vi "Pacemaker ASIC Test_Config Globals.vi"() -> ()   [LabVIEW 2016]
panel:
  in  "software version 2":string="build  2097"
  in  "software version 1":string="ASIC Test  V0.10.0.1"
  out "uut  note":string="IC_all"
  in  "id strings":string[][](table)
  out "note":string
  out "data time":string="20121102_163200"
  out "uut  sn":string="29A"
  out "uut version":string="03A"
  out "uut pn":string="MC20"
  in  "Shunt":T1={"Ib Vol"=1.0, "Ib Cur"=1e-08, "Ibat Vol"=0.007765, "Ibat Cur"=1e-06, "Load Vrega Vol"=-1.0, "Load Vrega Cur"=1e-05, "Load Vregd Vol"=-1.0, "Load Vregd Cur"=0.0002, "Load Vha Vol"=-1.0, "Load Vha Cur"=0.0002} {"Load Vha Cur" format="%#_6p"; "Load Vregd Cur" format="%#_6p"; "Load Vrega Cur" format="%#_6p"; "Ibat Cur" format="%#_6p"; "Ibat Vol" format="%#_6p"; "Ib Cur" format="%#_6p"; "Ib Vol" format="%#_6p"}
  out "TableReg":string[][](table)=[["Function_Name", "Bit_Name", "Data[B]", ""], ["System Control Register", "CPUOk", "0", ""], ["System Control Register", "RDSMASK", "0", ""], ["System Control Register", "LPWMASK", "0", ""], ["System Control Register", "TPSLEEP", "0", ""], ["System Control Register", "VUR", "0", ""], ["System Control Register", "VUT", "1", ""], ["System Control Register", "AUR", "0", ""], ["System Control Register", "AUT", "1", ""], ["Atrial Pulse Dutation Control Register", "ABILUNISEL", "1", ""], ["Atrial Pulse Dutation Control Register", "ARCHG[2]", "1", ""], ["Atrial Pulse Dutation Control Register", "ARCHG[1]", "0", ""], ["Atrial Pulse Dutation Control Register", "ARCHG[0]", "1", ""], ["Atrial Pulse Dutation Control Register", "APW[3]", "1", ""], ["Atrial Pulse Dutation Control Register", "APW[2]", "0", ""], ["Atrial Pulse Dutation Control Register", "APW[1]", "0", ""], ["Atrial Pulse Dutation Control Register", "APW[0]", "0", ""], ["Atrial Pace Amplitude Control Register", "APUMPGN[1]", "1", ""], ["Atrial Pace Amplitude Control Register", "APUMPGN[0]", "0", ""], ["Atrial Pace Amplitude Control Register", "APAMP[5]", "1", ""], ["Atrial Pace Amplitude Control Register", "APAMP[4]", "0", ""], ["Atrial Pace Amplitude Control Register", "APAMP[3]", "1", ""], ["Atrial Pace Amplitude Control Register", "APAMP[2]", "0", ""], ["Atrial Pace Amplitude Control Register", "APAMP[1]", "0", ""], ["Atrial Pace Amplitude Control Register", "APAMP[0]", "0", ""], ["Ventricular Pulse Duration Control Register", "VBILUNISEL", "1", ""], ["Ventricular Pulse Duration Control Register", "VRCHG[2]", "1", ""], ["Ventricular Pulse Duration Control Register", "VRCHG[1]", "0", ""], ["Ventricular Pulse Duration Control Register", "VRCHG[0]", "1", ""], ["Ventricular Pulse Duration Control Register", "VPW[3]", "1", ""], ["Ventricular Pulse Duration Control Register", "VPW[2]", "0", ""], ["Ventricular Pulse Duration Control Register", "VPW[1]", "0", ""], ["Ventricular Pulse Duration Control Register", "VPW[0]", "0", ""], ["Ventricular Pace Amplitude Control Register", "VPUMPGN[1]", "1", ""], ["Ventricular Pace Amplitude Control Register", "VPUMPGN[0]", "0", ""], ["Ventricular Pace Amplitude Control Register", "VPAMP[5]", "1", ""], ["Ventricular Pace Amplitude Control Register", "VPAMP[4]", "0", ""], ["Ventricular Pace Amplitude Control Register", "VPAMP[3]", "1", ""], ["Ventricular Pace Amplitude Control Register", "VPAMP[2]", "0", ""], ["Ventricular Pace Amplitude Control Register", "VPAMP[1]", "0", ""], ["Ventricular Pace Amplitude Control Register", "VPAMP[0]", "0", ""], ["Blank/Mask Control Register", "AAIFLG", "0", ""], ["Blank/Mask Control Register", "PVAB[4]", "0", ""], ["Blank/Mask Control Register", "PVAB[3]", "1", ""], ["Blank/Mask Control Register", "PVAB[2]", "0", ""], ["Blank/Mask Control Register", "PVAB[1]", "0", ""], ["Blank/Mask Control Register", "PVAB[0]", "1", ""], ["Blank/Mask Control Register", "OBLANK[1]", "1", ""], ["Blank/Mask Control Register", "OBLANK[0]", "1", ""], ["Atrial Sensitivity Control Register", "Spare", "0", ""], ["Atrial Sensitivity Control Register", "ASGN[1]", "1", ""], ["Atrial Sensitivity Control Register", "ASGN[0]", "1", ""], ["Atrial Sensitivity Control Register", "AS[4]", "0", ""], ["Atrial Sensitivity Control Register", "AS[3]", "1", ""], ["Atrial Sensitivity Control Register", "AS[2]", "0", ""], ["Atrial Sensitivity Control Register", "AS[1]", "0", ""], ["Atrial Sensitivity Control Register", "AS[0]", "1", ""], ["Ventricular Sensitivity Control Register", "Spare", "0", ""], ["Ventricular Sensitivity Control Register", "VSGN[1]", "0", ""], ["Ventricular Sensitivity Control Register", "VSGN[0]", "1", ""], ["Ventricular Sensitivity Control Register", "VS[4]", "0", ""], ["Ventricular Sensitivity Control Register", "VS[3]", "1", ""], ["Ventricular Sensitivity Control Register", "VS[2]", "1", ""], ["Ventricular Sensitivity Control Register", "VS[1]", "0", ""], ["Ventricular Sensitivity Control Register", "VS[0]", "1", ""], ["Measure Request Register", "Spare", "0", ""], ["Measure Request Register", "TPUMPEN", "0", ""], ["Measure Request Register", "EGMFS", "0", ""], ["Measure Request Register", "EGMREQ[1]", "0", ""], ["Measure Request Register", "EGMREQ[0]", "0", ""], ["Measure Request Register", "MREQ[2]", "0", ""], ["Measure Request Register", "MREQ[1]", "0", ""], ["Measure Request Register", "MREQ[0]", "0", ""], ["Measurement Result Register 1", "MRESULT1[7]", "0", ""], ["Measurement Result Register 1", "MRESULT1[6]", "0", ""], ["Measurement Result Register 1", "MRESULT1[5]", "0", ""], ["Measurement Result Register 1", "MRESULT1[4]", "0", ""], ["Measurement Result Register 1", "MRESULT1[3]", "0", ""], ["Measurement Result Register 1", "MRESULT1[2]", "0", ""], ["Measurement Result Register 1", "MRESULT1[1]", "0", ""], ["Measurement Result Register 1", "MRESULT1[0]", "0", ""], ["Measurement Result Register 2", "MRESULT2[7]", "0", ""], ["Measurement Result Register 2", "MRESULT2[6]", "0", ""], ["Measurement Result Register 2", "MRESULT2[5]", "0", ""], ["Measurement Result Register 2", "MRESULT2[4]", "0", ""], ["Measurement Result Register 2", "MRESULT2[3]", "0", ""], ["Measurement Result Register 2", "MRESULT2[2]", "0", ""], ["Measurement Result Register 2", "MRESULT2[1]", "0", ""], ["Measurement Result Register 2", "MRESULT2[0]", "0", ""], ["Telemetry Downlink Data Length Register", "Spare", "0", ""], ["Telemetry Downlink Data Length Register", "Spare", "0", ""], ["Telemetry Downlink Data Length Register", "RFDLEN2CPU[5]", "0", ""], ["Telemetry Downlink Data Length Register", "RFDLEN2CPU[4]", "0", ""], ["Telemetry Downlink Data Length Register", "RFDLEN2CPU[3]", "0", ""], ["Telemetry Downlink Data Length Register", "RFDLEN2CPU[2]", "0", ""], ["Telemetry Downlink Data Length Register", "RFDLEN2CPU[1]", "0", ""], ["Telemetry Downlink Data Length Register", "RFDLEN2CPU[0]", "0", ""], ["Telemetry Marker Low Byte Data Register", "MARKER2RF[7]", "0", ""], ["Telemetry Marker Low Byte Data Register", "MARKER2RF[6]", "0", ""], ["Telemetry Marker Low Byte Data Register", "MARKER2RF[5]", "0", ""], ["Telemetry Marker Low Byte Data Register", "MARKER2RF[4]", "0", ""], ["Telemetry Marker Low Byte Data Register", "MARKER2RF[3]", "0", ""], ["Telemetry Marker Low Byte Data Register", "MARKER2RF[2]", "0", ""], ["Telemetry Marker Low Byte Data Register", "MARKER2RF[1]", "0", ""], ["Telemetry Marker Low Byte Data Register", "MARKER2RF[0]", "0", ""], ["Telemetry Marker High Byte Data Register", "MARKER2RF[15]", "0", ""], ["Telemetry Marker High Byte Data Register", "MARKER2RF[14]", "0", ""], ["Telemetry Marker High Byte Data Register", "MARKER2RF[13]", "0", ""], ["Telemetry Marker High Byte Data Register", "MARKER2RF[12]", "0", ""], ["Telemetry Marker High Byte Data Register", "MARKER2RF[11]", "0", ""], ["Telemetry Marker High Byte Data Register", "MARKER2RF[10]", "0", ""], ["Telemetry Marker High Byte Data Register", "MARKER2RF[9]", "0", ""], ["Telemetry Marker High Byte Data Register", "MARKER2RF[8]", "0", ""], ["Telemetry Handshake Data Register", "RSW", "0", ""], ["Telemetry Handshake Data Register", "HSOK", "0", ""], ["Telemetry Handshake Data Register", "TPINSS", "0", ""], ["Telemetry Handshake Data Register", "TBD[4]", "0", ""], ["Telemetry Handshake Data Register", "TBD[3]", "0", ""], ["Telemetry Handshake Data Register", "TBD[2]", "0", ""], ["Telemetry Handshake Data Register", "TBD[1]", "0", ""], ["Telemetry Handshake Data Register", "TBD[0]", "0", ""], ["Telemetry Session ID Register", "SID2RF", "0", ""], ["Telemetry Session ID Register", "SID2RF", "0", ""], ["Telemetry Session ID Register", "SID2RF", "0", ""], ["Telemetry Session ID Register", "SID2RF", "0", ""], ["Telemetry Session ID Register", "SID2RF", "0", ""], ["Telemetry Session ID Register", "SID2RF", "0", ""], ["Telemetry Session ID Register", "SID2RF", "0", ""], ["Telemetry Session ID Register", "SID2RF", "0", ""], ["BIR Result Low Register", "BIRRESU[7]", "0", ""], ["BIR Result Low Register", "BIRRESU[6]", "0", ""], ["BIR Result Low Register", "BIRRESU[5]", "0", ""], ["BIR Result Low Register", "BIRRESU[4]", "0", ""], ["BIR Result Low Register", "BIRRESU[3]", "0", ""], ["BIR Result Low Register", "BIRRESU[2]", "0", ""], ["BIR Result Low Register", "BIRRESU[1]", "0", ""], ["BIR Result Low Register", "BIRRESU[0]", "0", ""], ["BIR Result High Register", "Spare", "0", ""], ["BIR Result High Register", "Spare", "0", ""], ["BIR Result High Register", "Spare", "0", ""], ["BIR Result High Register", "Spare", "0", ""], ["BIR Result High Register", "Spare", "0", ""], ["BIR Result High Register", "Spare", "0", ""], ["BIR Result High Register", "BIRRESU[9]", "0", ""], ["BIR Result High Register", "BIRRESU[8]", "0", ""], ["Pump Time Low Register", "TPUMP[7]", "0", ""], ["Pump Time Low Register", "TPUMP[6]", "0", ""], ["Pump Time Low Register", "TPUMP[5]", "0", ""], ["Pump Time Low Register", "TPUMP[4]", "0", ""], ["Pump Time Low Register", "TPUMP[3]", "0", ""], ["Pump Time Low Register", "TPUMP[2]", "0", ""], ["Pump Time Low Register", "TPUMP[1]", "0", ""], ["Pump Time Low Register", "TPUMP[0]", "0", ""], ["Pump Time High Register", "TPUMP[15]", "0", ""], ["Pump Time High Register", "TPUMP[14]", "0", ""], ["Pump Time High Register", "TPUMP[13]", "0", ""], ["Pump Time High Register", "TPUMP[12]", "0", ""], ["Pump Time High Register", "TPUMP[11]", "0", ""], ["Pump Time High Register", "TPUMP[10]", "0", ""], ["Pump Time High Register", "TPUMP[9]", "0", ""], ["Pump Time High Register", "TPUMP[8]", "0", ""], ["Measurement Control Register", "Spare", "0", ""], ["Measurement Control Register", "Spare", "0", ""], ["Measurement Control Register", "Spare", "0", ""], ["Measurement Control Register", "Spare", "0", ""], ["Measurement Control Register", "RLOFF", "1", ""], ["Measurement Control Register", "RK_SEL[2]", "0", ""], ["Measurement Control Register", "RK_SEL[1]", "0", ""], ["Measurement Control Register", "RK_SEL[0]", "0", ""], ["Trim RC32k Register", "Spare", "0", ""], ["Trim RC32k Register", "Spare", "0", ""], ["Trim RC32k Register", "TRIM_RC32k[5]", "1", ""], ["Trim RC32k Register", "TRIM_RC32k[4]", "0", ""], ["Trim RC32k Register", "TRIM_RC32k[3]", "0", ""], ["Trim RC32k Register", "TRIM_RC32k[2]", "0", ""], ["Trim RC32k Register", "TRIM_RC32k[1]", "0", ""], ["Trim RC32k Register", "TRIM_RC32k[0]", "0", ""], ["Trim RC1p6k Register", "Spare", "0", ""], ["Trim RC1p6k Register", "Spare", "0", ""], ["Trim RC1p6k Register", "TRIM_RC1P6K[5]", "1", ""], ["Trim RC1p6k Register", "TRIM_RC1P6K[4]", "0", ""], ["Trim RC1p6k Register", "TRIM_RC1P6K[3]", "0", ""], ["Trim RC1p6k Register", "TRIM_RC1P6K[2]", "0", ""], ["Trim RC1p6k Register", "TRIM_RC1P6K[1]", "0", ""], ["Trim RC1p6k Register", "TRIM_RC1P6K[0]", "0", ""], ["Trim VREGA Register", "Spare", "0", ""], ["Trim VREGA Register", "Spare", "0", ""], ["Trim VREGA Register", "Spare", "0", ""], ["Trim VREGA Register", "TRIM_VREGA[4]", "0", ""], ["Trim VREGA Register", "TRIM_VREGA[3]", "1", ""], ["Trim VREGA Register", "TRIM_VREGA[2]", "0", ""], ["Trim VREGA Register", "TRIM_VREGA[1]", "0", ""], ["Trim VREGA Register", "TRIM_VREGA[0]", "1", ""], ["Trim VREGD Register", "Spare", "0", ""], ["Trim VREGD Register", "Spare", "0", ""], ["Trim VREGD Register", "ENOBLP2", "0", ""], ["Trim VREGD Register", "TRIM_VREGD[4]", "0", ""], ["Trim VREGD Register", "TRIM_VREGD[3]", "1", ""], ["Trim VREGD Register", "TRIM_VREGD[2]", "0", ""], ["Trim VREGD Register", "TRIM_VREGD[1]", "0", ""], ["Trim VREGD Register", "TRIM_VREGD[0]", "1", ""], ["Trim LPF HPF Register", "TRIM_HPFBW[3]", "1", ""], ["Trim LPF HPF Register", "TRIM_HPFBW[2]", "0", ""], ["Trim LPF HPF Register", "TRIM_HPFBW[1]", "0", ""], ["Trim LPF HPF Register", "TRIM_HPFBW[0]", "0", ""], ["Trim LPF HPF Register", "TRIM_LPFBW[3]", "1", ""], ["Trim LPF HPF Register", "TRIM_LPFBW[2]", "0", ""], ["Trim LPF HPF Register", "TRIM_LPFBW[1]", "0", ""], ["Trim LPF HPF Register", "TRIM_LPFBW[0]", "0", ""], ["Trim IBIAS Register", "ENCASES", "1", ""], ["Trim IBIAS Register", "CSVEN", "1", ""], ["Trim IBIAS Register", "CSAEN", "1", ""], ["Trim IBIAS Register", "TRIM_IBIAS[4]", "0", ""], ["Trim IBIAS Register", "TRIM_IBIAS[3]", "1", ""], ["Trim IBIAS Register", "TRIM_IBIAS[2]", "0", ""], ["Trim IBIAS Register", "TRIM_IBIAS[1]", "0", ""], ["Trim IBIAS Register", "TRIM_IBIAS[0]", "0", ""], ["Trim IBIPT Register", "ENOBHP", "1", ""], ["Trim IBIPT Register", "ENOBLP1", "0", ""], ["Trim IBIPT Register", "DOBEN", "1", ""], ["Trim IBIPT Register", "TRIM_IBIPT[4]", "1", ""], ["Trim IBIPT Register", "TRIM_IBIPT[3]", "0", ""], ["Trim IBIPT Register", "TRIM_IBIPT[2]", "0", ""], ["Trim IBIPT Register", "TRIM_IBIPT[1]", "0", ""], ["Trim IBIPT Register", "TRIM_IBIPT[0]", "0", ""], ["Trim Band Gap Voltage Register", "TBIRON", "0", ""], ["Trim Band Gap Voltage Register", "TBIRON", "0", ""], ["Trim Band Gap Voltage Register", "MASKN", "0", ""], ["Trim Band Gap Voltage Register", "TRIM_BANDGAPV[4]", "0", ""], ["Trim Band Gap Voltage Register", "TRIM_BANDGAPV[3]", "1", ""], ["Trim Band Gap Voltage Register", "TRIM_BANDGAPV[2]", "0", ""], ["Trim Band Gap Voltage Register", "TRIM_BANDGAPV[1]", "0", ""], ["Trim Band Gap Voltage Register", "TRIM_BANDGAPV[0]", "1", ""], ["Digital Test Signal Select Register", "Spare", "0", ""], ["Digital Test Signal Select Register", "Spare", "0", ""], ["Digital Test Signal Select Register", "Spare", "0", ""], ["Digital Test Signal Select Register", "DTO_SEL[4]", "0", ""], ["Digital Test Signal Select Register", "DTO_SEL[3]", "0", ""], ["Digital Test Signal Select Register", "DTO_SEL[2]", "0", ""], ["Digital Test Signal Select Register", "DTO_SEL[1]", "0", ""], ["Digital Test Signal Select Register", "DTO_SEL[0]", "0", ""], ["Analog Switch Control Register", "ExSenseEn", "0", ""], ["Analog Switch Control Register", "Test_sel_b[3]", "0", ""], ["Analog Switch Control Register", "Test_sel_b[2]", "0", ""], ["Analog Switch Control Register", "Test_sel_b[1]", "0", ""], ["Analog Switch Control Register", "Test_sel_b[0]", "0", ""], ["Analog Switch Control Register", "Test_sel_a[2]", "0", ""], ["Analog Switch Control Register", "Test_sel_a[1]", "0", ""], ["Analog Switch Control Register", "Test_sel_a[0]", "0", ""], ["Test Control Register 1", "CPEN", "1", ""], ["Test Control Register 1", "FBCMEN", "1", ""], ["Test Control Register 1", "NHSTENV", "0", ""], ["Test Control Register 1", "NHSTENA", "0", ""], ["Test Control Register 1", "PDSV2", "1", ""], ["Test Control Register 1", "PDSA2", "1", ""], ["Test Control Register 1", "PDSV1", "0", ""], ["Test Control Register 1", "PDSA1", "0", ""], ["Test Control Register 2", "Spare", "0", ""], ["Test Control Register 2", "Spare", "0", ""], ["Test Control Register 2", "Spare", "0", ""], ["Test Control Register 2", "AntDigtest", "1", ""], ["Test Control Register 2", "ANTENN", "0", ""], ["Test Control Register 2", "ENWD", "0", ""], ["Test Control Register 2", "RC1P6KEN", "1", ""], ["Test Control Register 2", "RC32KEN", "0", ""], ["Telemetry Message or Downlink Data Buffer", "TPBUF64", "0", ""], ["Telemetry Message or Downlink Data Buffer", "TPBUF64", "0", ""], ["Telemetry Message or Downlink Data Buffer", "TPBUF64", "0", ""], ["Telemetry Message or Downlink Data Buffer", "TPBUF64", "0", ""], ["Telemetry Message or Downlink Data Buffer", "TPBUF64", "0", ""], ["Telemetry Message or Downlink Data Buffer", "TPBUF64", "0", ""], ["Telemetry Message or Downlink Data Buffer", "TPBUF64", "0", ""], ["Telemetry Message or Downlink Data Buffer", "TPBUF64", "0", ""], ["", "", "", ""], ["", "", "", ""], ["", "", "", ""], ["", "", "", ""], ["", "", "", ""], ["", "", "", ""], ["", "", "", ""], ["", "", "", ""], ["", "", "", ""], ["", "", "", ""], ["", "", "", ""], ["", "", "", ""], ["", "", "", ""], ["", "", "", ""], ["", "", "", ""], ["", "", "", ""], ["", "", "", ""], ["", "", "", ""], ["", "", "", ""], ["", "", "", ""], ["", "", "", ""], ["", "", "", ""], ["", "", "", ""], ["", "", "", ""], ["", "", "", ""], ["", "", "", ""], ["", "", "", ""]]
  out "TableRelay":string[][](table)
  in  "AWG":refnum<visa-resource-name>="GPIB0::10::INSTR"
  in  "Register":refnum<visa-resource-name>="COM1"
  in  "SPI DIO Channels":cluster{"CS":tag, "SCL":tag, "SO":tag, "SI":tag}={"CS"="6259/port0/line3", "SCL"="6259/port0/line0", "SO"="6259/port0/line1", "SI"="6259/port0/line2"}
  in  "595 DIO Channels":cluster{"SH_CP":tag, "DS":tag, "ST_CP":tag}={"SH_CP"="6259B/port0/line1", "DS"="6259B/port0/line6", "ST_CP"="6259B/port0/line4"}
  in  "Angilent Scope":refnum<visa-resource-name>="MSO7014A"
  in  "Temp Controller":refnum<visa-resource-name>="COM1"
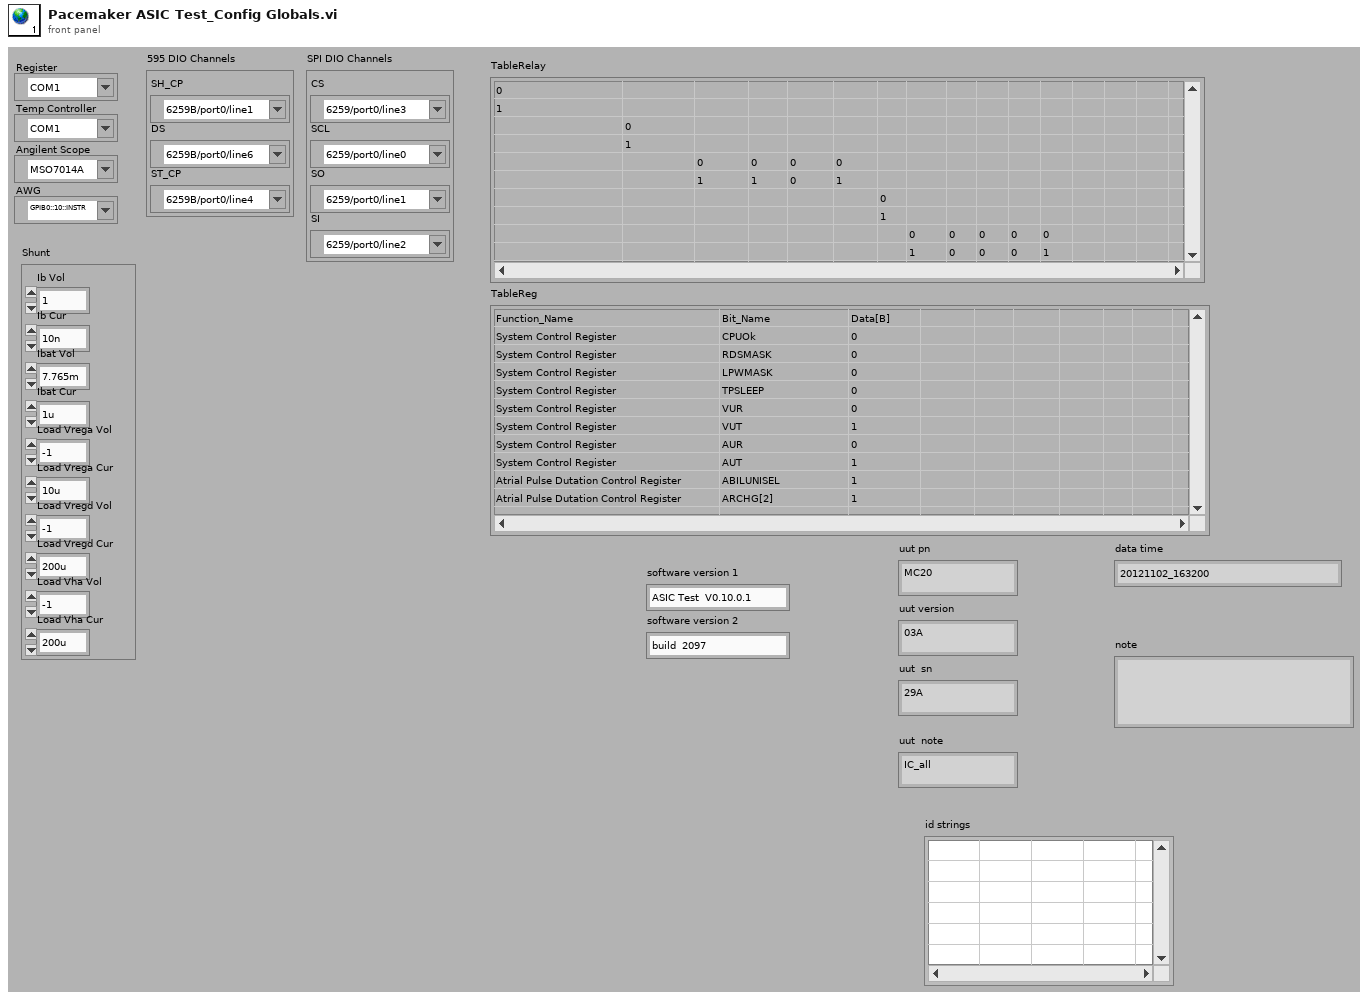
[diagram p1: front panel]
types:
  T1 = cluster{"Ib Vol":dbl, "Ib Cur":dbl, "Ibat Vol":dbl, "Ibat Cur":dbl, "Load Vrega Vol":dbl, "Load Vrega Cur":dbl, "Load Vregd Vol":dbl, "Load Vregd Cur":dbl, "Load Vha Vol":dbl, "Load Vha Cur":dbl}
diagram:
